vi "DHE_SendStat.vi"(9 "Message":string) -> ()   [LabVIEW 2016]
uses:
  DBSHAND/private/vis/DatabaseHand_Element_Get(string).vi
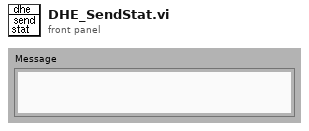
[diagram p1: front panel]
types:
  T1 = typedef "DatabaseHand_RefNum.ctl" = refnum<vi>
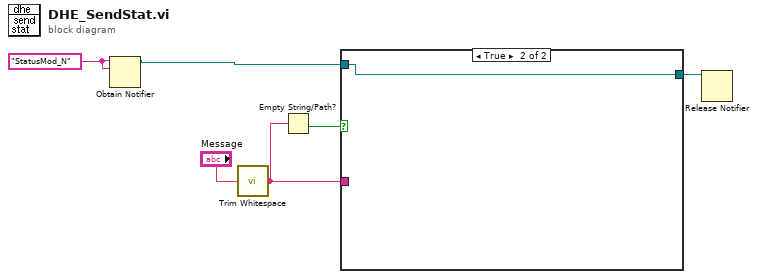
[diagram p0: block diagram]
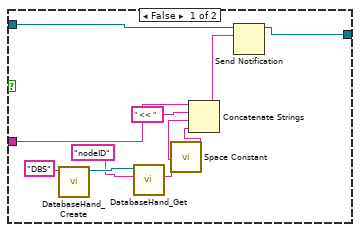
[diagram p2: hidden frame]
diagram:
  w3 = "StatusMod_N" ("name (unnamed)")
  n1 = Obtain Notifier(name (unnamed)=w3, notification data type=w3) -> (notifier out=w2:refnum<notifier>)  [unwired: 2 in, 2 out]
  n2 = call <vilib>:"Trim Whitespace.vi"("string"="Message") -> ("trimmed string"=w5:string)  [unwired: 1 in]
  n3 = Empty String/Path?(string/path=w5) -> (empty?=w4:bool)
  n4 = case shown="True" w4 {
    tunnel: w5 -> [w15 _]
    tunnel: w2 -> [w14 w17]
    tunnel: [w7 w17] -> w1
    frame False {
      n5 = call "DatabaseHand_Create.vi"("Name"="DBS") -> ("Database RefNum out"=w12:T1)  [unwired: 1 in, 9 out]
      n6 = call-poly "DatabaseHand_Get.vi"("name"="nodeID", "Database RefNum in"=w12) -> ("value"=w9:string)  [unwired: 3 in, 6 out]
      n7 = call <vilib>:"Space Constant.vi"() -> ("String"=w8:string)
      n8 = Concatenate Strings(w15, " << " ("string"), w9, w8) -> (w16:string)
      n9 = Send Notification(notification=w16, notifier=w14) -> (notifier out=w7:refnum<notifier>)  [unwired: 1 in, 1 out]
    }
    frame True {
    }
  }
  n10 = Release Notifier(notifier=w1) -> ()  [unwired: 1 in, 4 out]
